vi "Post Launch Init.vi"(8 "error in":errorcluster, 11 "Report Generator in":refnum<class "Report Generator.lvclass">) -> (0 "error out":errorcluster, 3 "Report Generator out":refnum<class "Report Generator.lvclass">, 4 "Events":T1, 6 "Self Enqueuer":refnum<class "Message Enqueuer.lvclass">)   [LabVIEW 2019, in "Report Generator.lvlib" / "Report Generator.lvclass"]
uses:
  Library/Report Generator.lvclass
  C:/Users/Public/Documents/Development/builds/Engine/Engine.lvlibp/Project/Engine.lvclass
  builds/Engine/Actor Framework.lvlibp/1abvi3w/vi.lib/ActorFramework/Message Enqueuer/Message Enqueuer.lvclass
  builds/Engine/Panel.lvlibp/Panel Helper/Panel Events.ctl
  builds/Engine/Panel.lvlibp/Panel Helper/Events.ctl
  builds/Engine/Engine.lvlibp/Custom Controls/System Events.ctl
  builds/Engine/Engine.lvlibp/Custom Controls/System Status.ctl
  builds/Engine/Engine.lvlibp/Custom Controls/Manual Events.ctl
  builds/Engine/Engine.lvlibp/Custom Controls/UUT_Events.ctl
  builds/Engine/Engine.lvlibp/Accessors/Read Events.vi
  builds/Engine/Panel Manager.lvlibp/Panel Actor/Panel Actor.lvclass
  C:/Users/Public/Documents/Development/builds/Engine/Panel Manager.lvlibp/Panel Actor/Panel Actor.lvclass
  builds/Engine/Panel.lvlibp/Panel Helper/Panel Helper.lvclass
  builds/Engine/Engine.lvlibp/Project/Engine.lvclass
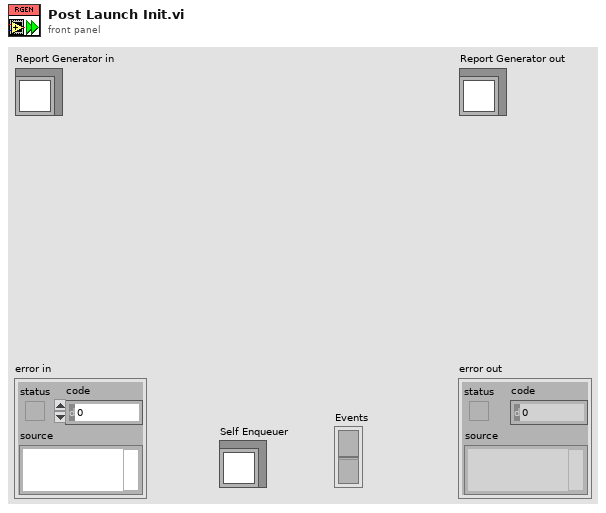
[diagram p1: front panel]
types:
  T1 = cluster{"Pnl Actor":refnum<event-registration>, "Event Registration Refnum":refnum<event-registration>}
  T2 = typedef "Engine.lvlibp/Engine.lvclass/Engine Events.ctl" = cluster{"System Event":T3, "Manual":T4, "UUT":T5, "Interface Events":T6}
  T3 = typedef "Engine.lvlibp/Engine.lvclass/System Events.ctl" = cluster{"Fault Event":refnum<user-event>, "SystemStatus Event":refnum<user-event>, "Automation":refnum<user-event>}
  T4 = typedef "Engine.lvlibp/Engine.lvclass/Manual Events.ctl" = cluster{"QuickStart Event":refnum<user-event>, "SafeBTE Event":refnum<user-event>, "TogglePower Event":refnum<user-event>, "Change Instrument Event":refnum<user-event>, "Toggle Launch Event":refnum<user-event>, "UUTSupply":refnum<user-event>}
  T5 = typedef "Engine.lvlibp/Engine.lvclass/UUT_Events.ctl" = cluster{"UUT_Name":refnum<user-event>, "Test_Name":refnum<user-event>, "Test_Operator":refnum<user-event>, "Test_Witness":refnum<user-event>, "Pedigree_Event":refnum<user-event>}
  T6 = typedef "Engine.lvlibp/Engine.lvclass/Interface Events.ctl" = cluster{"Interface_Command":refnum<user-event>, "Telemetry_Descriptor":refnum<user-event>, "AsynchTLM_Descriptor":refnum<user-event>}
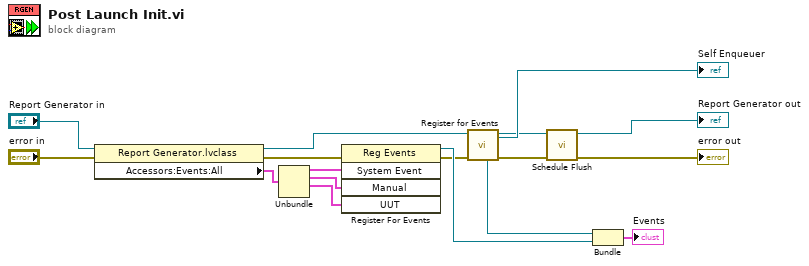
[diagram p0: block diagram]
diagram:
  n1 = property class="Report Generator.lvclass"(reference="Report Generator in", error in="error in") -> (reference out=w16:refnum<class "Report Generator.lvclass">, error out=w11:errorcluster, "Accessors:Events:All"=w5:T2)
  n2 = Unbundle(w5) -> ("System Event"=w4:T3, "Manual"=w3:T4, "UUT"=w2:T5)  [unwired: 1 out]
  n3 = register-events(error in=w11, w4, w3, w2) -> (reference out=w14:refnum<event-registration>, error out=w10:errorcluster)  [unwired: 1 in]
  n4 = call "Register for Events.vi"("Error In"=w10, "Panel Actor in"=w16) -> ("Error Out"=w8:errorcluster, "Panel Actor out"=w9:refnum<class "Report Generator.lvclass">, "Pnl Actor"=w15:refnum<event-registration>, "Self Enqueuer"=→"Self Enqueuer":refnum<class "Message Enqueuer.lvclass">)  [unwired: 6 in]
  n5 = call "Schedule Flush.vi"("error in"=w8, "Report Generator in"=w9) -> ("error out"=→"error out":errorcluster, "Report Generator out"=→"Report Generator out":refnum<class "Report Generator.lvclass">)  [unwired: 8 in]
  n6 = Bundle("Pnl Actor"=w15, "Event Registration Refnum"=w14) -> (→"Events":T1)  [unwired: 1 in]
